vi "OneBallAuto.vi"() -> ()   [LabVIEW 2020]
uses:
  Global Variables/AutoOneBall.ctl
  <vilib>/Rock Robotics/WPI/ThirdParty/REV Robotics/REVLib/Typedef/Spark MAX Control Type.ctl
  Global Variables/ActuatorsSensors.vi
  Global Variables/Axes_N_Buttons.vi
panel:
  out "PID R":cluster{"Sensor Position":dbl, "Setpoint":dbl}(graph)
  out "PID L":cluster{"Sensor Position":dbl, "Setpoint":dbl}(graph)
  in  "PID Constants R":T1={"P Gain"=0.0, "I Gain"=0.0, "D Gain"=0.0, "F Gain"=0.0, "I Zone"=0.0, "Min Output"=-1.0, "Max Output"=1.0}
  in  "PID Constants L":T1={"P Gain"=0.0, "I Gain"=0.0, "D Gain"=0.0, "F Gain"=0.0, "I Zone"=0.0, "Min Output"=-1.0, "Max Output"=1.0}
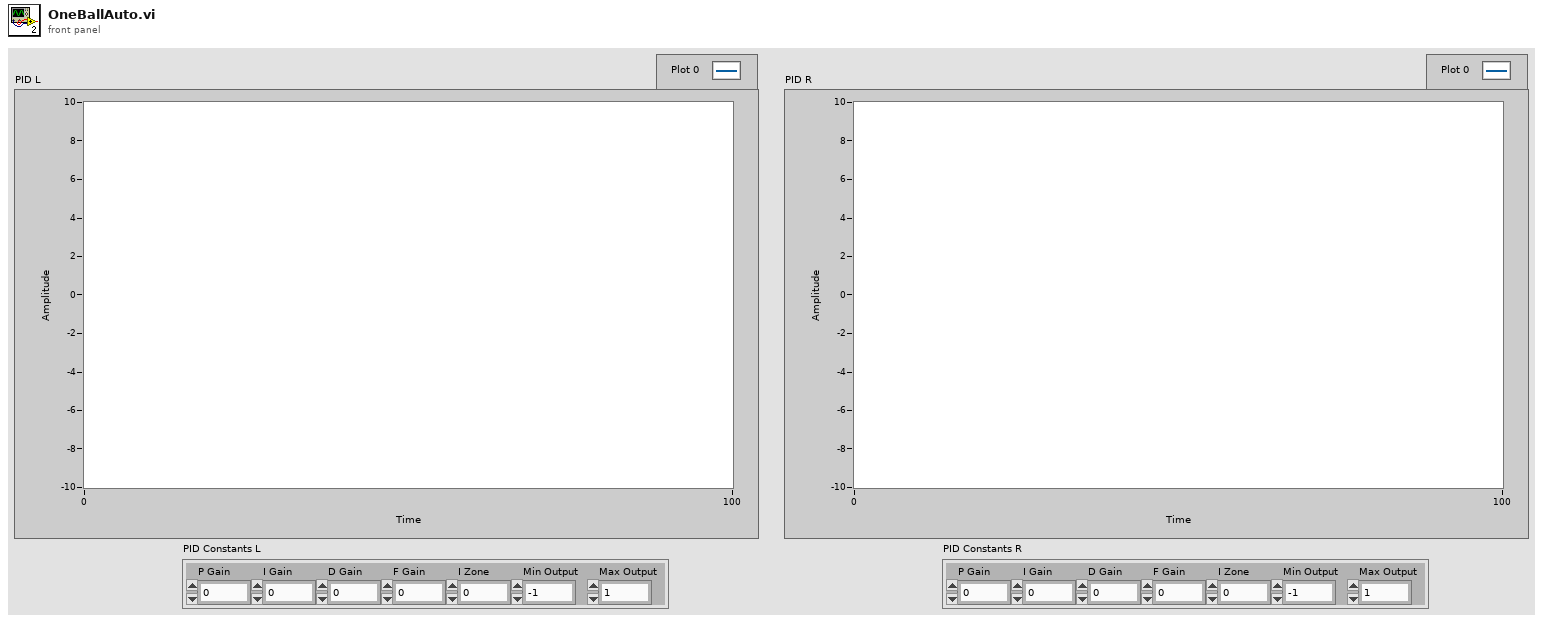
[diagram p1: front panel]
types:
  T1 = cluster{"P Gain":dbl, "I Gain":dbl, "D Gain":dbl, "F Gain":dbl, "I Zone":dbl, "Min Output":dbl, "Max Output":dbl}
  T2 = typedef "AutoOneBall.ctl" = enum16{"Start", "Shoot", "Delay", "Exit Tarmac", "Reset"}
  T3 = typedef "WPI_MotorControlDeviceRef.ctl" = cluster{"DeviceStatus":errorcluster, "Type":T4, "PWM":cluster{"PWM Channel":T5, "DeadBand":T6}, "CAN":cluster{"Device Number":u8, "SetOutput VI Ref":variant, "GetOutput VI Ref":variant, "Enable VI Ref":variant, "Disable VI Ref":variant, "Data":variant}, "Invert":bool, "DIO PWM":cluster{"PWM \"Enable\" Channel":T5, "DIOChannel":T7, "PWM Rate":dbl}}
  T4 = typedef "WPI_MotorControlType.ctl" = enum16{"PWM", "CAN", "DIO PWM"}
  T5 = typedef "FPGA_DIOPWMChannel.ctl" = enum8{"PWM 0", "PWM 1", "PWM 2", "PWM 3", "PWM 4", "PWM 5", "PWM 6", "PWM 7", "PWM 8", "PWM 9", "PWM MXP 0", "PWM MXP 1", "PWM MXP 2", "PWM MXP 3", "PWM MXP 4", "PWM MXP 5", "PWM MXP 6", "PWM MXP 7", "PWM MXP 8", "PWM MXP 9", "Invalid"}
  T6 = typedef "WPI_PWMDeadband.ctl" = cluster{"Name":string, "maxPositivePwm":i32, "minPositivePwm":i32, "centerPwm":i32, "maxNegativePwm":i32, "minNegativePwm":i32, "angularRange":u16}
  T7 = typedef "FPGA_DIOChannel.ctl" = enum8{"DIO 0", "DIO 1", "DIO 2", "DIO 3", "DIO 4", "DIO 5", "DIO 6", "DIO 7", "DIO 8", "DIO 9", "DIO MXP 0", "DIO MXP 1", "DIO MXP 2", "DIO MXP 3", "DIO MXP 4", "DIO MXP 5", "DIO MXP 6", "DIO MXP 7", "DIO MXP 8", "DIO MXP 9", "DIO MXP 10", "DIO MXP 11", "DIO MXP 12", "DIO MXP 13", "DIO MXP 14", "DIO MXP 15", "SPI Port CS1", "SPI Port CS2", "SPI Port CS3", "SPI Port MISO", "SPI Port MOSI", "Invalid"}
  T8 = typedef "Spark MAX Control Type.ctl" = enum16{"Percent VBus", "Voltage", "Velocity", "Position", "Smart Motion", "Current", "Smart Velocity"}
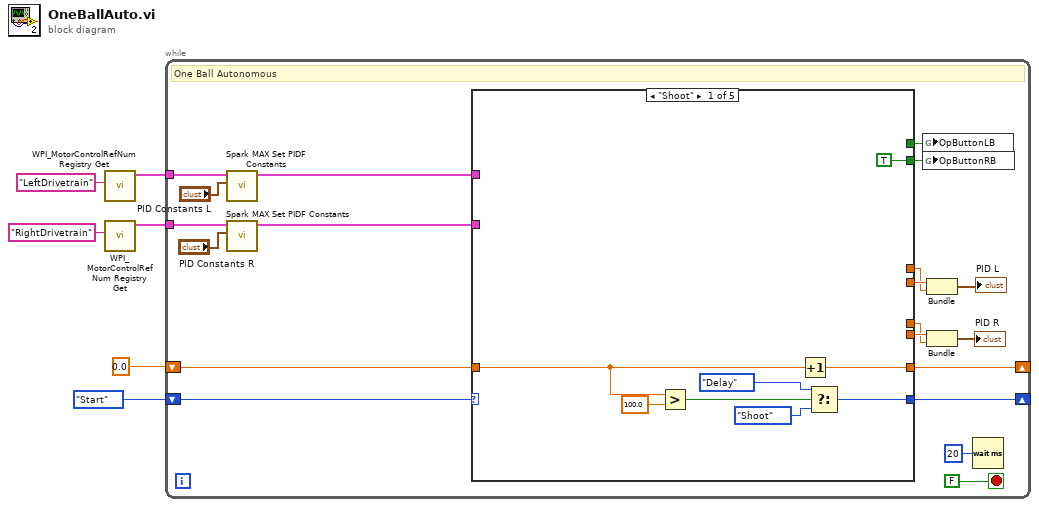
[diagram p0: block diagram]
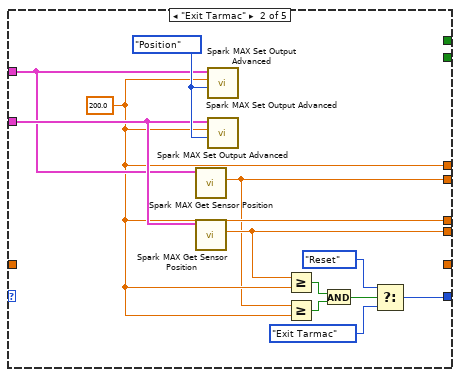
[diagram p2: hidden frame]
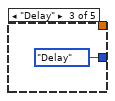
[diagram p3: hidden frame]
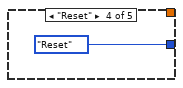
[diagram p4: hidden frame]
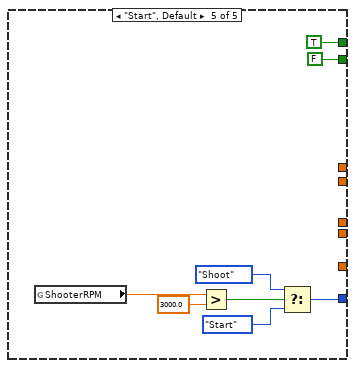
[diagram p5: hidden frame]
diagram:
  n1 = call <vilib>:"WPI_MotorControlRefNum Registry Get.vi"("refnum name"="LeftDrivetrain") -> ("MotorControlDevRef"=w3:T3)  [unwired: 9 in, 1 out]
  n2 = call <vilib>:"WPI_MotorControlRefNum Registry Get.vi"("refnum name"="RightDrivetrain") -> ("MotorControlDevRef"=w2:T3)  [unwired: 9 in, 1 out]
  n3 = while {
    shift-right: [w18] -> _
    shift-left: AutoOneBall."Start" ("Enum") -> [w26]
    tunnel: w3 -> [w22]
    tunnel: w2 -> [w23]
    shift-right: [w7] -> _
    shift-left: 0.0 ("Setpoint") -> [w8]
    stop <- FALSE stop-if-true
    # "One Ball Autonomous"
    n4 = call <vilib>:"Spark MAX Set PIDF Constants.vi"("PID Constants"="PID Constants L", "MotorControlDeviceRef"=w22) -> ("MotorControlDeviceRef"=w20:T3)  [unwired: 8 in, 1 out]
    n5 = call <vilib>:"Spark MAX Set PIDF Constants.vi"("PID Constants"="PID Constants R", "MotorControlDeviceRef"=w23) -> ("MotorControlDeviceRef"=w21:T3)  [unwired: 8 in, 1 out]
    n6 = case shown="\"Shoot\"" w26 {
      tunnel: w21 -> [_ w45 _ _ _]
      tunnel: w20 -> [_ w44 _ _ _]
      tunnel: [_ _ _ _ TRUE ("OpButtonLB")] -> w19
      tunnel: [w27 w35 AutoOneBall."Delay" ("Enum") AutoOneBall."Reset" ("Enum") w50] -> w18
      tunnel: [_ w41 _ _ _] -> w15
      tunnel: [_ w43 _ _ _] -> w14
      tunnel: [_ w42 _ _ _] -> w13
      tunnel: [_ w42 _ _ _] -> w12
      tunnel: [TRUE ("DrButtonRB") _ _ _ FALSE ("DrButtonRB")] -> w9
      tunnel: w8 -> [w33 _ _ _ _]
      tunnel: [w31 _ _ _ _] -> w7
      frame "Shoot" {
        n7 = Greater?(x=w33, y=100.0) -> (0:w30:bool)
        n8 = Increment(x=w33) -> (x+1=w31:dbl)
        n9 = Select(t=AutoOneBall."Delay" ("Enum"), s=w30, f=AutoOneBall."Shoot" ("Enum")) -> (s? t:f=w27:T2)
      }
      frame "Exit Tarmac" {
        w42 = 200.0 ("Setpoint")
        w46 = Spark_MAX_Control_Type."Position" ("Control Mode")
        n10 = call <vilib>:"Spark MAX Get Sensor Position.vi"("MotorControlDevRef in"=w44) -> ("Sensor Position"=w41:dbl)  [unwired: 7 in, 3 out]
        n11 = call <vilib>:"Spark MAX Get Sensor Position.vi"("MotorControlDevRef in"=w45) -> ("Sensor Position"=w43:dbl)  [unwired: 7 in, 3 out]
        n12 = call <vilib>:"Spark MAX Set Output Advanced.vi"("Control Mode"=w46, "Setpoint"=w42, "MotorControlDevRef"=w44) -> ()  [unwired: 7 in, 2 out]
        n13 = call <vilib>:"Spark MAX Set Output Advanced.vi"("Control Mode"=w46, "Setpoint"=w42, "MotorControlDevRef"=w44) -> ()  [unwired: 7 in, 2 out]
        n14 = call <vilib>:"Spark MAX Set Output Advanced.vi"("Control Mode"=w46, "Setpoint"=w42, "MotorControlDevRef"=w45) -> ()  [unwired: 7 in, 2 out]
        n15 = Greater Or Equal?(x=w43, y=w42) -> (x >= y?=w40:bool)
        n16 = Greater Or Equal?(x=w41, y=w42) -> (x >= y?=w39:bool)
        n17 = And(x=w40, y=w39) -> (x .and. y?=w38:bool)
        n18 = Select(t=AutoOneBall."Reset" ("Enum"), s=w38, f=AutoOneBall."Exit Tarmac" ("Enum")) -> (s? t:f=w35:T2)
      }
      frame "Delay" {
      }
      frame "Reset" {
      }
      frame "Start", Default {
        n19 = global read "ActuatorsSensors.vi" "ShooterRPM"() -> (w55:dbl)
        n20 = Greater?(x=w55, y=3000.0) -> (0:w53:bool)
        n21 = Select(t=AutoOneBall."Shoot" ("Enum"), s=w53, f=AutoOneBall."Start" ("Enum")) -> (s? t:f=w50:T2)
      }
    }
    n22 = global write "Axes_N_Buttons.vi" "OpButtonLB"(w19) -> ()
    n23 = global write "Axes_N_Buttons.vi" "OpButtonRB"(w9) -> ()
    n24 = Bundle("Sensor Position"=w15, "Setpoint"=w13) -> (→"PID L":cluster{"Sensor Position":dbl, "Setpoint":dbl})  [unwired: 1 in]
    n25 = Bundle("Sensor Position"=w14, "Setpoint"=w12) -> (→"PID R":cluster{"Sensor Position":dbl, "Setpoint":dbl})  [unwired: 1 in]
    n26 = Wait (ms)(milliseconds to wait=u32 20) -> ()  [unwired: 1 out]
  }
